vi "Filter Data.vi"(8 "error in (no error)":errorcluster, 10 "Debug Data In":refnum<class "Debug Data.lvclass">[](array[class]), 11 "Mock Filter in":refnum<class "Mock Filter.lvclass">) -> (0 "error out":errorcluster, 2 "Debug Data Out":refnum<class "Debug Data.lvclass">[](array[class]), 3 "Mock Filter out":refnum<class "Mock Filter.lvclass">)   [LabVIEW 2020, in "Mock Filter.lvclass"]
uses:
  Mock Filter.lvclass
  Debug Data/Debug Data.lvclass
  Mock Filter.lvclass/Mock Filter.ctl
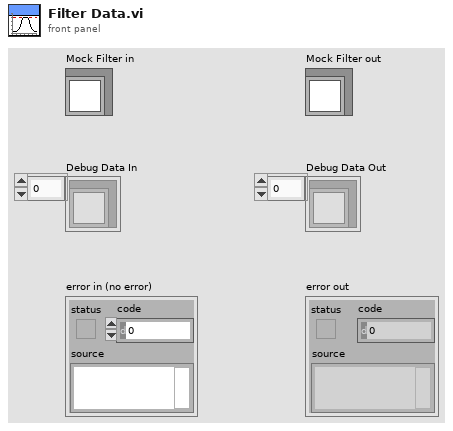
[diagram p1: front panel]
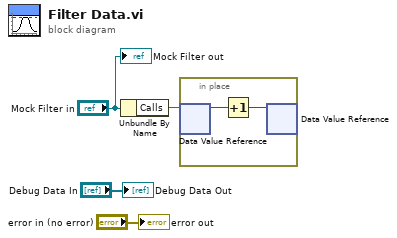
[diagram p0: block diagram]
diagram:
  n1 = Unbundle By Name("Mock Filter in") -> ("Calls"=w2:refnum<data-value>)
  n2 = in-place {
    n3 = in-place-dvr #1(w2) -> (w6:i32)  [unwired: 1 out]
    n4 = Increment(x=w6) -> (x+1=w5:i32)
    n5 = in-place-dvr #1(w5) -> ()  [unwired: 2 out]
  }
  "error out" <- "error in (no error)"
  "Mock Filter out" <- "Mock Filter in"
  "Debug Data Out" <- "Debug Data In"
